vi "Write Data.vi"(8 "error in (no error)":errorcluster, 10 "Anything":variant, 11 "ITransport in":refnum<class "ITransport.lvclass">) -> (0 "error out":errorcluster, 3 "ITransport out":refnum<class "ITransport.lvclass">)   [LabVIEW 2015, in "Mediator.lvlib" / "ITransport.lvclass"]
uses:
  ITransport.lvclass
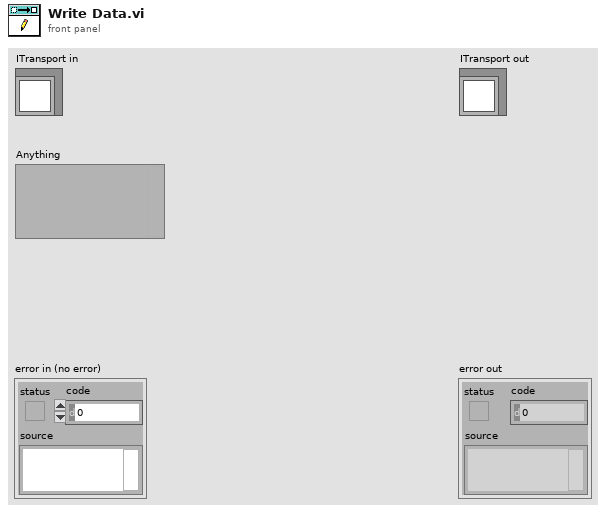
[diagram p1: front panel]
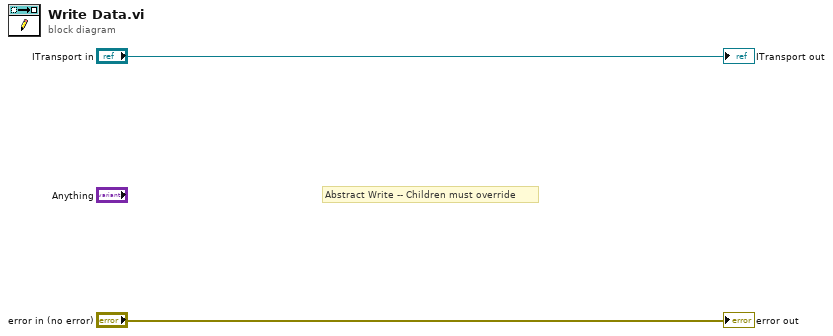
[diagram p0: block diagram]
diagram:
  # "Abstract Write -- Children must override"
  "error out" <- "error in (no error)"
  "ITransport out" <- "ITransport in"
